vi "Open Shorts Test.vi"(10 "All Pins":string[](array[string]), 11 "Semiconductor Module Context":T1) -> (0 "error out":errorcluster)   [LabVIEW 2013]
uses:
  <vilib>/NI_TestStand_SemiconductorModule/NI_TestStand_Semiconductor_Module.lvlibp/PinMap/General/SemiconductorModuleContext.ctl
  <vilib>/NI_TestStand_SemiconductorModule/NI_TestStand_Semiconductor_Module.lvlibp/PinMap/General/NIInstrumentTypeIDs.ctl
  <instrlib>/niDCPower/nidcpower.llb/niDCPower Wait For Event - Event.ctl
  <instrlib>/niDCPower/nidcpower.llb/niDCPower Output Function.ctl
  <instrlib>/niHSDIO/niHSDIO.llb/niHSDIO_ctl stPMU Sense Terminal.ctl
  <instrlib>/niHSDIO/niHSDIO.llb/niHSDIO_ctl stPMU Disable Return State.ctl
  <vilib>/NI_TestStand_SemiconductorModule/NI_TestStand_Semiconductor_Module.lvlibp/PinMap/DC Power/PinsToNIDCPowerSessions.vi
  <vilib>/NI_TestStand_SemiconductorModule/NI_TestStand_Semiconductor_Module.lvlibp/PinMap/HSDIO/PinsToNIHSDIOSessions.vi
  <vilib>/NI_TestStand_SemiconductorModule/NI_TestStand_Semiconductor_Module.lvlibp/PinMap/General/Publish/PublishDataDouble2D.vi
  <vilib>/NI_TestStand_SemiconductorModule/NI_TestStand_Semiconductor_Module.lvlibp
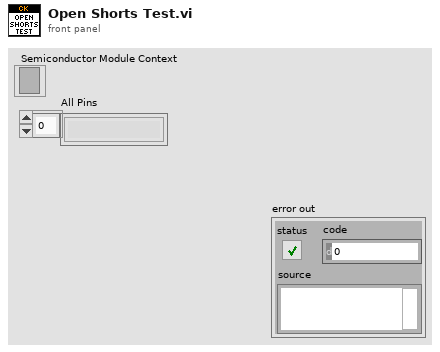
[diagram p1: front panel]
types:
  T1 = typedef "NI_TestStand_Semiconductor_Module.lvlibp/SemiconductorModuleContext.ctl" = refnum<k7>
  T2 = typedef "NI_TestStand_Semiconductor_Module.lvlibp/NIInstrumentTypeIDs.ctl" = string
  T3 = typedef "niDCPower Output Function.ctl" = i32
  T4 = typedef "niDCPower Wait For Event - Event.ctl" = i32
  T5 = typedef "niHSDIO_ctl stPMU Sense Terminal.ctl" = i32
  T6 = typedef "niHSDIO_ctl stPMU Disable Return State.ctl" = u32
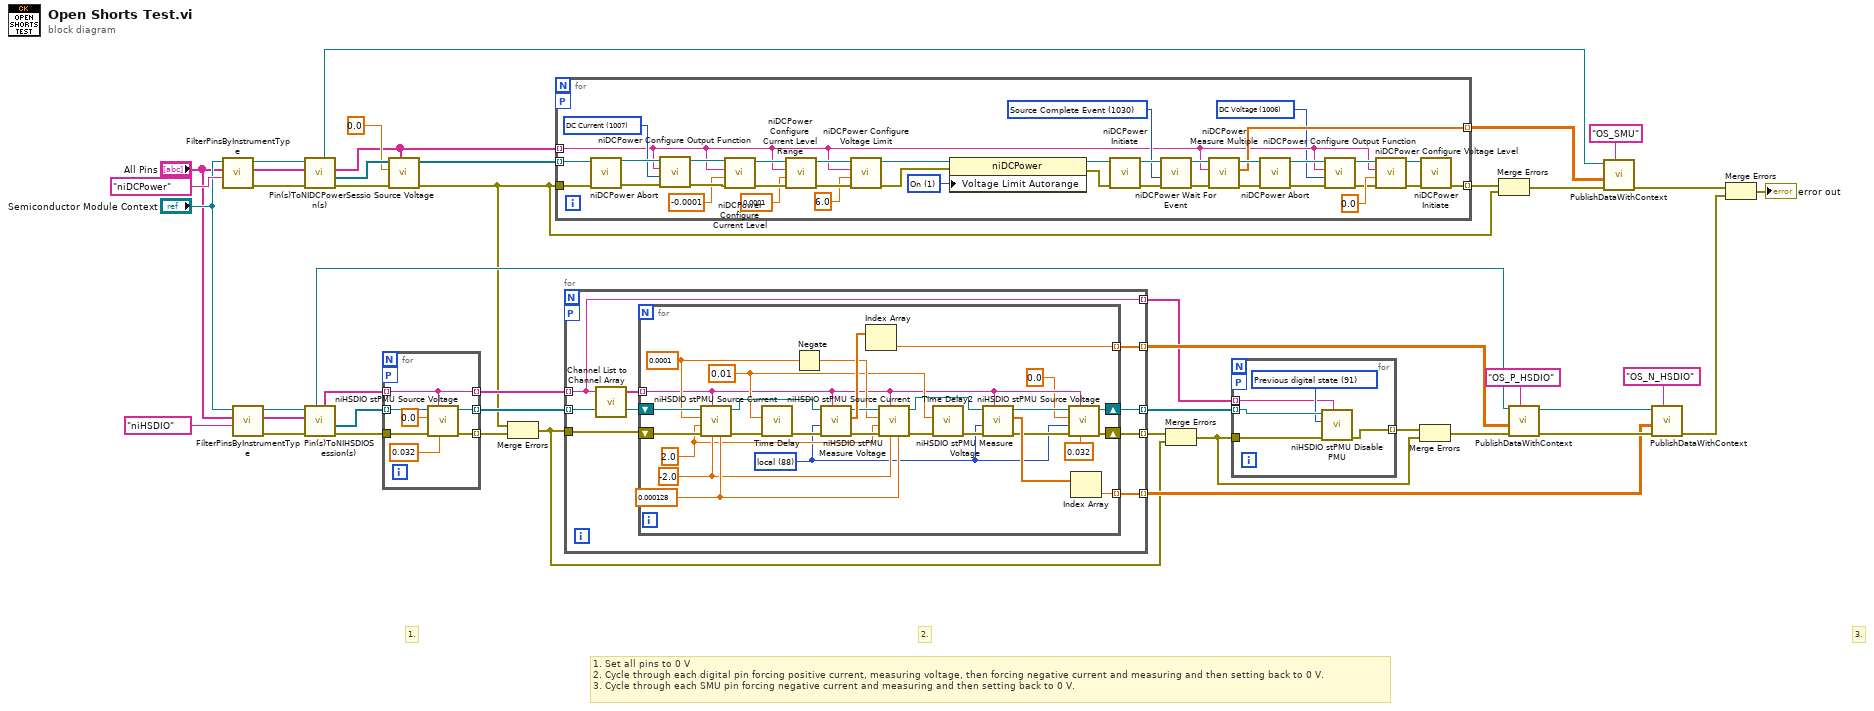
[diagram p0: block diagram]
diagram:
  # "1. Set all pins to 0 V\n2. Cycle through each digital pin forcing positive current, measuring voltage, then forcing negative current and measuring and then setting back to 0 V.\n3. Cycle through each SMU pin forcing negative current and measuring and then setting back to 0 V."
  # "3."
  # "2."
  # "1."
  n1 = call <vilib>:"FilterPinsByInstrumentType.vi"("Instrument Type Id"=T2 "niDCPower", "Pins"="All Pins", "Semiconductor Module Context"="Semiconductor Module Context") -> ("error out"=w40:errorcluster, "Filtered Pins"=w1:string[], "Semiconductor Module Context Out"=w39:T1)  [unwired: 6 in]
  n2 = call <vilib>:"FilterPinsByInstrumentType.vi"("Instrument Type Id"=T2 "niHSDIO", "Pins"="All Pins", "Semiconductor Module Context"="Semiconductor Module Context") -> ("error out"=w38:errorcluster, "Filtered Pins"=w21:string[], "Semiconductor Module Context Out"=w37:T1)  [unwired: 6 in]
  n3 = call-poly <vilib>:"Pin(s)ToNIDCPowerSession(s).vi"("error in (no error)"=w40, "Pins"=w1, "Semiconductor Module Context"=w39) -> ("error out"=w44:errorcluster, "Instrument Sessions"=w43:refnum<k15>[], "Channel Lists"=w19:string[], "Pin Query Context"=w4:refnum<class "MultiplePinMultipleSessionQueryContext.lvclass">)  [unwired: 4 in, 1 out]
  n4 = call-poly <vilib>:"Pin(s)ToNIHSDIOSession(s).vi"("error in (no error)"=w38, "Pins"=w21, "Semiconductor Module Context"=w37) -> ("error out"=w33:errorcluster, "Generation Sessions"=w32:refnum<k15>[], "Channel Lists"=w31:string[], "Pin Query Context"=w5:refnum<class "MultiplePinMultipleSessionQueryContext.lvclass">)  [unwired: 3 in, 2 out]
  n5 = for {
    tunnel: w33 -> [w51]
    tunnel: w32 -> [w50] mode=indexing
    tunnel: w31 -> [w45] mode=indexing
    tunnel: [w47] -> w30 mode=indexing
    tunnel: [w46] -> w29 mode=indexing
    tunnel: [w45] -> w28 mode=indexing
    workers-P: _ -> [_]
    n6 = call <instrlib>:"niHSDIO stPMU Source Voltage.vi"("current range"=0.032, "channel list"=w45, "error in (no error)"=w51, "voltage level"=0.0, "instrument handle"=w50) -> ("error out"=w47:errorcluster, "instrument handle out"=w46:refnum<k15>)  [unwired: 5 in]
  }
  n7 = call "Source Voltage.vi"("Channel Lists"=w19, "error in (no error)"=w44, "voltage level"=0.0, "Instrument Sessions In"=w43) -> ("error out"=w3:errorcluster, "Instrument Sessions Out"=w20:refnum<k15>[])  [unwired: 4 in, 2 out]
  n8 = Merge Errors(w3, w30) -> (w9:errorcluster)
  n9 = for {
    tunnel: w20 -> [w87] mode=indexing
    tunnel: w19 -> [w55] mode=indexing
    tunnel: [w70] -> w17 mode=indexing
    tunnel: w3 -> [w88]
    tunnel: [w72] -> w8 mode=indexing
    workers-P: _ -> [_]
    w54 = T3 1006 items=["DC Voltage"=1006, "DC Current"=1007, "Pulse Voltage"=1049, "Pulse Current"=1050] ("output function")
    w60 = T3 1007 items=["DC Voltage"=1006, "DC Current"=1007, "Pulse Voltage"=1049, "Pulse Current"=1050] ("output function")
    w67 = T4 1030 items=["Source Complete Event"=1030, "Measure Complete Event"=1031, "Sequence Iteration Complete Event"=1032, "Sequence Engine Done Event"=1033, "Pulse Complete Event"=1051, "Ready For Pulse Trigger Event"=1052] ("event")
    w81 = 1 items=["Off", "On"] ("Source:DC Current:Voltage Limit Autorange")
    n10 = call <instrlib>:"niDCPower Abort.vi"("error in (no error)"=w88, "instrument handle"=w87) -> ("error out"=w64:errorcluster, "instrument handle out"=w63:refnum<k15>)  [unwired: 8 in]
    n11 = call <instrlib>:"niDCPower Configure Output Function.vi"("error in (no error)"=w64, "output function"=w60, "channel name"=w55, "instrument handle"=w63) -> ("error out"=w62:errorcluster, "instrument handle out"=w61:refnum<k15>)  [unwired: 6 in]
    n12 = call <instrlib>:"niDCPower Configure Current Level.vi"("error in (no error)"=w62, "current level"=-0.0001, "channel name"=w55, "instrument handle"=w61) -> ("error out"=w86:errorcluster, "instrument handle out"=w85:refnum<k15>)  [unwired: 6 in]
    n13 = call <instrlib>:"niDCPower Configure Current Level Range.vi"("error in (no error)"=w86, "current level range"=0.0001 ("current level"), "channel name"=w55, "instrument handle"=w85) -> ("error out"=w84:errorcluster, "instrument handle out"=w83:refnum<k15>)  [unwired: 6 in]
    n14 = call <instrlib>:"niDCPower Configure Voltage Limit.vi"("error in (no error)"=w84, "voltage limit"=6.0, "channel name"=w55, "instrument handle"=w83) -> ("error out"=w79:errorcluster, "instrument handle out"=w80:refnum<k15>)  [unwired: 6 in]
    n15 = property class="niDCPower"(reference=w80, error in=w79, "Voltage Limit Autorange"=w81) -> (reference out=w78:refnum<k15>, error out=w77:errorcluster)
    n16 = call <instrlib>:"niDCPower Initiate.vi"("error in (no error)"=w77, "instrument handle"=w78) -> ("error out"=w69:errorcluster, "instrument handle out"=w68:refnum<k15>)  [unwired: 8 in]
    n17 = call <instrlib>:"niDCPower Wait For Event.vi"("error in (no error)"=w69, "event"=w67, "instrument handle"=w68) -> ("error out"=w66:errorcluster, "instrument handle out"=w65:refnum<k15>)  [unwired: 7 in]
    n18 = call <instrlib>:"niDCPower Measure Multiple.vi"("error in (no error)"=w66, "channel name"=w55, "instrument handle"=w65) -> ("error out"=w76:errorcluster, "voltage measurements"=w70:dbl[], "instrument handle out"=w75:refnum<k15>)  [unwired: 5 in, 1 out]
    n19 = call <instrlib>:"niDCPower Abort.vi"("error in (no error)"=w76, "instrument handle"=w75) -> ("error out"=w59:errorcluster, "instrument handle out"=w58:refnum<k15>)  [unwired: 8 in]
    n20 = call <instrlib>:"niDCPower Configure Output Function.vi"("error in (no error)"=w59, "output function"=w54, "channel name"=w55, "instrument handle"=w58) -> ("error out"=w57:errorcluster, "instrument handle out"=w56:refnum<k15>)  [unwired: 6 in]
    n21 = call <instrlib>:"niDCPower Configure Voltage Level.vi"("error in (no error)"=w57, "voltage level"=0.0, "channel name"=w55, "instrument handle"=w56) -> ("error out"=w73:errorcluster, "instrument handle out"=w71:refnum<k15>)  [unwired: 6 in]
    n22 = call <instrlib>:"niDCPower Initiate.vi"("error in (no error)"=w73, "instrument handle"=w71) -> ("error out"=w72:errorcluster)  [unwired: 8 in, 1 out]
  }
  n23 = for {
    tunnel: w29 -> [w95] mode=indexing
    tunnel: w9 -> [w94]
    tunnel: w28 -> [w89] mode=indexing
    tunnel: [w93] -> w26 mode=indexing
    tunnel: [w92] -> w22 mode=indexing
    tunnel: [w91] -> w13 mode=indexing
    tunnel: [w90] -> w27 mode=indexing
    tunnel: [w89] -> w10 mode=indexing
    workers-P: _ -> [_]
    n24 = call "Channel List to Channel Array.vi"("Channel List"=w89) -> ("Channel Array"=w96:string[])  [unwired: 4 in]
    n25 = for {
      tunnel: w96 -> [w100] mode=indexing
      tunnel: [w118] -> w93 mode=indexing
      shift-right: [w102] -> w90
      shift-left: w94 -> [w124]
      tunnel: [w105] -> w92 mode=indexing
      shift-right: [w101] -> w91
      shift-left: w95 -> [w123]
      w98 = T5 88 items=["local"=88, "remote"=89] ("sense (local)")
      w109 = 0.01 ("Delay Time (s)")
      w113 = 0.000128 ("current range")
      w112 = -2.0 ("lower voltage limit")
      w111 = 2.0 ("upper voltage limit")
      w115 = 0.0001 ("current level")
      n26 = call <instrlib>:"niHSDIO stPMU Source Current.vi"("current range"=w113, "lower voltage limit"=w112, "channel list"=w100, "error in (no error)"=w124, "upper voltage limit"=w111, "current level"=w115, "instrument handle"=w123) -> ("error out"=w122:errorcluster, "instrument handle out"=w120:refnum<k15>)  [unwired: 3 in]
      n27 = call "Time Delay"("error in (no error)"=w122, "Delay Time (s)"=w109) -> ("error out"=w121:errorcluster)  [unwired: 9 in]
      n28 = Negate(x=w115) -> (-x=w114:dbl)
      n29 = call <instrlib>:"niHSDIO stPMU Measure Voltage.vi"("channel list"=w100, "error in (no error)"=w121, "sense (local)"=w98, "instrument handle"=w120) -> ("error out"=w117:errorcluster, "voltage measurements"=w119:dbl[], "instrument handle out"=w116:refnum<k15>)  [unwired: 5 in]
      n30 = Index Array(array=w119) -> (element=w118:dbl)  [unwired: 1 in]
      n31 = call <instrlib>:"niHSDIO stPMU Source Current.vi"("current range"=w113, "lower voltage limit"=w112, "channel list"=w100, "error in (no error)"=w117, "upper voltage limit"=w111, "current level"=w114, "instrument handle"=w116) -> ("error out"=w110:errorcluster, "instrument handle out"=w107:refnum<k15>)  [unwired: 3 in]
      n32 = call "Time Delay2"("error in (no error)"=w110, "Delay Time (s)"=w109) -> ("error out"=w108:errorcluster)  [unwired: 9 in]
      n33 = call <instrlib>:"niHSDIO stPMU Measure Voltage.vi"("channel list"=w100, "error in (no error)"=w108, "sense (local)"=w98, "instrument handle"=w107) -> ("error out"=w104:errorcluster, "voltage measurements"=w106:dbl[], "instrument handle out"=w103:refnum<k15>)  [unwired: 5 in]
      n34 = call <instrlib>:"niHSDIO stPMU Source Voltage.vi"("current range"=0.032, "channel list"=w100, "error in (no error)"=w104, "sense (local)"=w98, "voltage level"=0.0, "instrument handle"=w103) -> ("error out"=w102:errorcluster, "instrument handle out"=w101:refnum<k15>)  [unwired: 4 in]
      n35 = Index Array(array=w106) -> (element=w105:dbl)  [unwired: 1 in]
    }
  }
  n36 = Merge Errors(w27, w9) -> (w2:errorcluster)
  n37 = for {
    tunnel: w2 -> [w129]
    tunnel: w13 -> [w128] mode=indexing
    tunnel: [w126] -> w12 mode=indexing
    tunnel: w10 -> [w125] mode=indexing
    workers-P: _ -> [_]
    w127 = T6 91 items=["Tristate"=90, "Previous digital state"=91] ("return state (tristate)")
    n38 = call <instrlib>:"niHSDIO stPMU Disable PMU.vi"("channel list"=w125, "error in (no error)"=w129, "return state (tristate)"=w127, "instrument handle"=w128) -> ("error out"=w126:errorcluster)  [unwired: 6 in, 1 out]
  }
  n39 = Merge Errors(w12, w2) -> (w11:errorcluster)
  n40 = Merge Errors(w8, w3) -> (w7:errorcluster)
  n41 = call-poly <vilib>:"PublishDataWithContext.vi"("Published Data Id"="OS_P_HSDIO" ("Measurement Id"), "error in (no error)"=w11, "Data In"=w26, "Pin Query Context"=w5) -> ("error out"=w25:errorcluster, "Pin Query Context Out"=w6:refnum<class "MultiplePinMultipleSessionQueryContext.lvclass">)  [unwired: 6 in]
  n42 = call-poly <vilib>:"PublishDataWithContext.vi"("Published Data Id"="OS_SMU" ("Measurement Id"), "error in (no error)"=w7, "Data In"=w17, "Pin Query Context"=w4) -> ("error out"=w16:errorcluster)  [unwired: 6 in, 1 out]
  n43 = call-poly <vilib>:"PublishDataWithContext.vi"("Published Data Id"="OS_N_HSDIO" ("Measurement Id"), "error in (no error)"=w25, "Data In"=w22, "Pin Query Context"=w6) -> ("error out"=w15:errorcluster)  [unwired: 6 in, 1 out]
  n44 = Merge Errors(w16, w15) -> (→"error out":errorcluster)
